vi "AI N Samples FPGA（Host）.vi"() -> ()   [LabVIEW 2019]
uses:
  <vilib>/LabVIEW Targets/FPGA/RIO/BlueMoonOnboardIO/nicrio_cRIO-BlueMoonOnboardAi_VoltageRange.ctl
  <vilib>/LabVIEW Targets/FPGA/RIO/BlueMoonOnboardIO/nicrio_cRIO-BlueMoonOnboardAi_TerminalMod.ctl
  <vilib>/FPGAPlugInAG/ELVIS III/niLvFpga_Open_ELVIS III.vi
  <vilib>/rvi/interface/common/dynamic/niFpgaDynamicAddResources.vi
  <vilib>/rvi/interface/common/niFpgaWaitOnOcc.vi
  <vilib>/Utility/error.llb/Error Cluster From Error Code.vi
  <vilib>/rvi/errors/niLvFpgaAdjustHostInterfaceError.vi
  <vilib>/FPGAPlugInAG/Dynamic/niLvFpga_Run_Dynamic.vi
  <vilib>/FPGAPlugInAG/Dynamic/niLvFpga_Close_Dynamic.vi
  <vilib>/rvi/interface/nirviOpenFPGA/nirviOpenFPGA.xnode
  FPGA Bitfiles/analogio-fpga_FPGATarget_AINSamplesFPGA_QNEx0wyFWIE.lvbitx
  AI N Samples FPGA.vi
  <vilib>/rvi/interface/nirviMethod/nirviMethod.xnode
  <vilib>/rvi/interface/nirviReadWriteControl/nirviReadWriteControl.xnode
  <vilib>/rvi/interface/nirviCloseFPGA/nirviCloseFPGA.xnode
  <vilib>/FPGAPlugInAG/Dynamic/niLvFpga_ConfigureFifo_Dynamic.vi
  <vilib>/rvi/errors/niLvFpgaMergeErrorWithErrorCode.vi
  NiFpgaLv.dll
  <vilib>/rvi/interface/Simulation/niFpgaSimulationCallBeginRW.vi
  <vilib>/FPGAPlugInAG/Dynamic/niLvFpga_ReadFifo_Dynamic.vi
panel:
  in  "停止":bool
  out "波形图表":dbl[](graph)
  in  "A?B":bool=TRUE
  in  "Sample Number":u32=1000 format="%.0p"
  in  "Channel Number [i + 1]":u8
  in  "Terminal Mode [i + 1]":T1=1 items=["DIFF", "RSE"]
  in  "Voltage Range [i + 1]":T2 items=["+/- 10V", "+/- 5V", "+/- 2V", "+/- 1V"]
  in  "Sample Rate":u32=10000 format="%.0p"
  in  "Start":bool
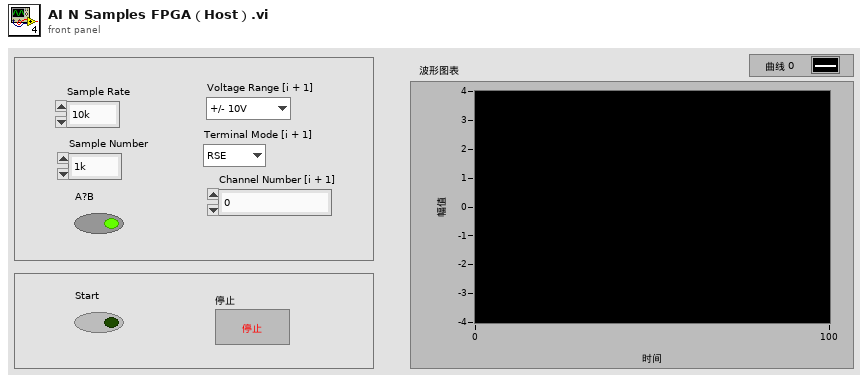
[diagram p1: front panel]
types:
  T1 = typedef "nicrio_cRIO-BlueMoonOnboardAi_TerminalMod.ctl" = u8
  T2 = typedef "nicrio_cRIO-BlueMoonOnboardAi_VoltageRange.ctl" = u8
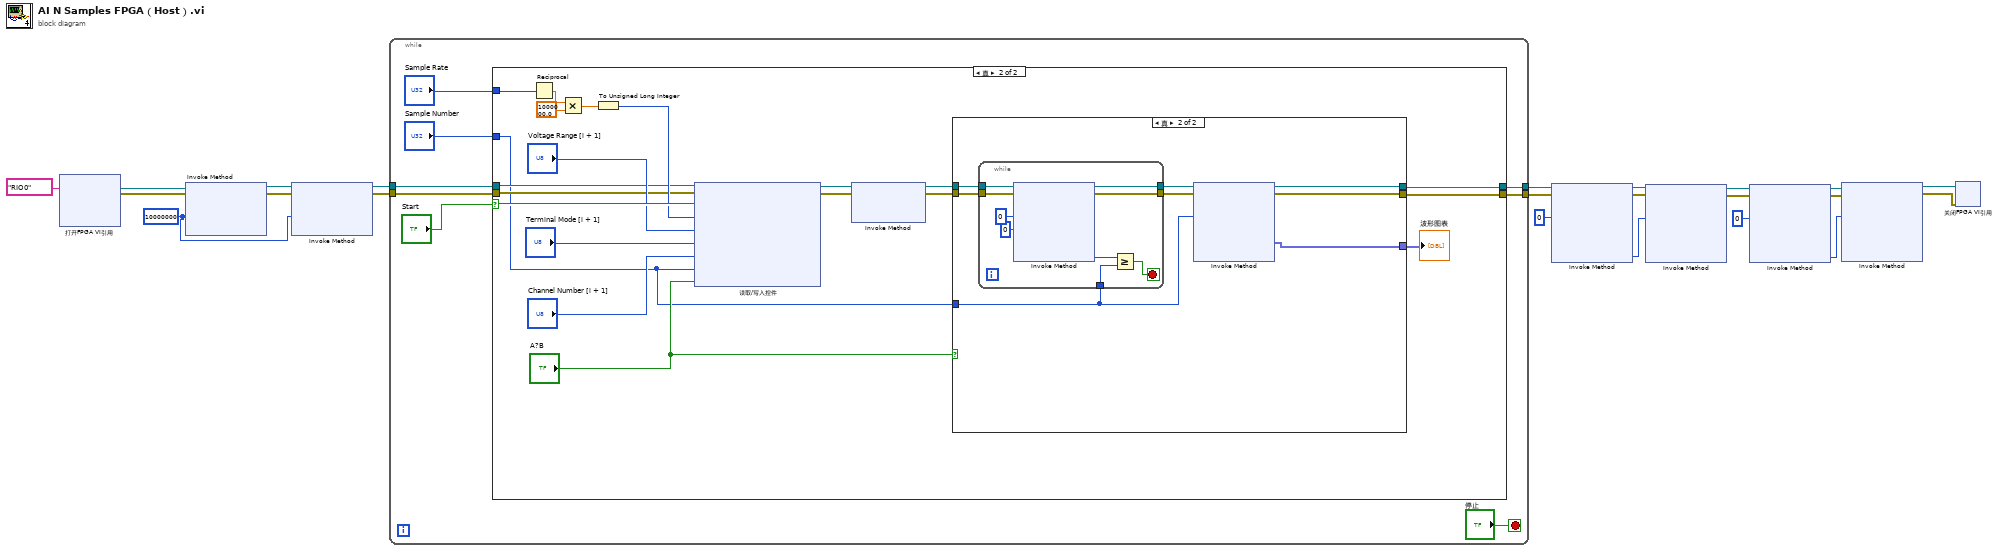
[diagram p0: block diagram]
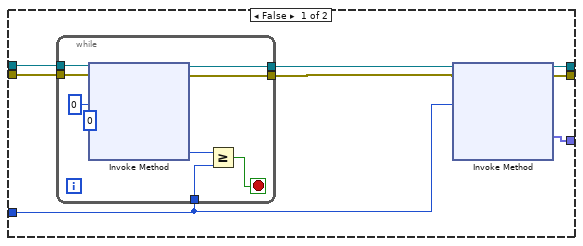
[diagram p3: hidden frame]
diagram:
  w17 = u32 10000000 ("请求的深度")
  n1 = xnode "打开FPGA VI引用"("资源名称"=tag "RIO0") -> ("FPGA VI引用输出"=w21:refnum<k20>, "错误输出"=w22:errorcluster)  [unwired: 1 in]
  n2 = xnode "Invoke Method"("FPGA VI引用输入"=w21, "错误输入"=w22, "请求的深度"=w17) -> ("FPGA VI引用输出"=w18:refnum<k20>, "错误输出"=w19:errorcluster)  [unwired: 1 out]
  n3 = xnode "Invoke Method"("FPGA VI引用输入"=w18, "错误输入"=w19, "请求的深度"=w17) -> ("FPGA VI引用输出"=w1:refnum<k20>, "错误输出"=w2:errorcluster)  [unwired: 1 out]
  n4 = while {
    tunnel: w2 -> [w28]
    tunnel: w1 -> [w29]
    tunnel: [w27] -> w16
    tunnel: [w26] -> w15
    stop <- "停止" stop-if-true
    n5 = case shown="真" "Start" {
      selector: "Start" -> [_ w48]
      tunnel: "Sample Number" -> [_ w40]
      tunnel: "Sample Rate" -> [_ w52]
      tunnel: w29 -> [w31 w42]
      tunnel: w28 -> [w32 w43]
      tunnel: [w32 w38] -> w27
      tunnel: [w31 w37] -> w26
      frame False {
      }
      frame True {
        n6 = Reciprocal(x=w52) -> (1/x=w51:dbl)
        n7 = Multiply(x=w51, y=1000000.0) -> (x*y=w49:dbl)
        n8 = To Unsigned Long Integer(number=w49) -> (unsigned 32bit integer=w44:u32)
        n9 = xnode "读取/写入控件"("FPGA VI引用输入"=w42, "错误输入"=w43, "Start"=w48, "Sample time"=w44, "Voltage Range [i + 1]"="Voltage Range [i + 1]", "Terminal Mode [i + 1]"="Terminal Mode [i + 1]", "Channel Number [i + 1]"="Channel Number [i + 1]", "Sample Number"=w40, "A?B"="A?B") -> ("FPGA VI引用输出"=w35:refnum<k20>, "错误输出"=w36:errorcluster)
        n10 = xnode "Invoke Method"("FPGA VI引用输入"=w35, "错误输入"=w36) -> ("FPGA VI引用输出"=w33:refnum<k20>, "错误输出"=w34:errorcluster)  [unwired: 1 in]
        n11 = case shown="真" "A?B" {
          tunnel: w34 -> [w59 w77]
          tunnel: w33 -> [w60 w76]
          tunnel: w40 -> [w58 w73]
          tunnel: [w57 w72] -> w39
          tunnel: [w56 w71] -> w38
          tunnel: [w55 w70] -> w37
          frame False {
            n12 = while {
              tunnel: w60 -> [w69]
              tunnel: w59 -> [w68]
              tunnel: w58 -> [w62]
              tunnel: [w67] -> w54
              tunnel: [w66] -> w53
              stop <- w61 stop-if-true
              n13 = xnode "Invoke Method"("FPGA VI引用输入"=w69, "错误输入"=w68, "元素数量"=u32 0, "超时(ms)"=0) -> ("FPGA VI引用输出"=w66:refnum<k20>, "错误输出"=w67:errorcluster, "剩余元素"=w63:u32)  [unwired: 1 out]
              n14 = Greater Or Equal?(x=w63, y=w62) -> (x >= y?=w61:bool)
            }
            n15 = xnode "Invoke Method"("FPGA VI引用输入"=w53, "错误输入"=w54, "元素数量"=w58) -> ("FPGA VI引用输出"=w55:refnum<k20>, "错误输出"=w56:errorcluster, "数据"=w57:fxp<+/-,24,5>[])  [unwired: 1 in, 1 out]
          }
          frame True {
            n16 = while {
              tunnel: w77 -> [w86]
              tunnel: w76 -> [w85]
              tunnel: w73 -> [w79]
              tunnel: [w83] -> w75
              tunnel: [w82] -> w74
              stop <- w78 stop-if-true
              n17 = xnode "Invoke Method"("FPGA VI引用输入"=w85, "错误输入"=w86, "元素数量"=u32 0, "超时(ms)"=0) -> ("FPGA VI引用输出"=w82:refnum<k20>, "错误输出"=w83:errorcluster, "剩余元素"=w80:u32)  [unwired: 1 out]
              n18 = Greater Or Equal?(x=w80, y=w79) -> (x >= y?=w78:bool)
            }
            n19 = xnode "Invoke Method"("FPGA VI引用输入"=w74, "错误输入"=w75, "元素数量"=w73) -> ("FPGA VI引用输出"=w70:refnum<k20>, "错误输出"=w71:errorcluster, "数据"=w72:fxp<+/-,24,5>[])  [unwired: 1 in, 1 out]
          }
        }
        "波形图表" <- w39
      }
    }
  }
  n20 = xnode "Invoke Method"("FPGA VI引用输入"=w15, "错误输入"=w16, "元素数量"=u32 0) -> ("FPGA VI引用输出"=w13:refnum<k20>, "错误输出"=w12:errorcluster, "剩余元素"=w11:u32)  [unwired: 1 in, 1 out]
  n21 = xnode "Invoke Method"("FPGA VI引用输入"=w13, "错误输入"=w12, "元素数量"=w11) -> ("FPGA VI引用输出"=w10:refnum<k20>, "错误输出"=w9:errorcluster)  [unwired: 1 in, 2 out]
  n22 = xnode "Invoke Method"("FPGA VI引用输入"=w10, "错误输入"=w9, "元素数量"=u32 0) -> ("FPGA VI引用输出"=w6:refnum<k20>, "错误输出"=w7:errorcluster, "剩余元素"=w5:u32)  [unwired: 1 in, 1 out]
  n23 = xnode "Invoke Method"("FPGA VI引用输入"=w6, "错误输入"=w7, "元素数量"=w5) -> ("FPGA VI引用输出"=w4:refnum<k20>, "错误输出"=w3:errorcluster)  [unwired: 1 in, 2 out]
  n24 = xnode "关闭FPGA VI引用"("FPGA VI引用输入"=w4, "错误输入"=w3) -> ()  [unwired: 1 out]
